vi "get-stage-positions.vi"(8 "error in (no error)":errorcluster, 11 "Cluster":T2) -> (0 "error out":errorcluster, 3 "stage positions":T1)   [LabVIEW 2024]
uses:
  C:/Users/hpDIRC/Desktop/eic_dirc_daq-LabVIEW_new/Thorlabs/Thorlabs.MotionControl.IntegratedStepperMotorsCLI.dll
  Thorlabs/Thorlabs.MotionControl.IntegratedStepperMotorsCLI.dll
  C:/Users/hpDIRC/Desktop/eic_dirc_daq-LabVIEW_new/Thorlabs/Thorlabs.MotionControl.Benchtop.StepperMotorCLI.dll
  Thorlabs/Thorlabs.MotionControl.Benchtop.StepperMotorCLI.dll
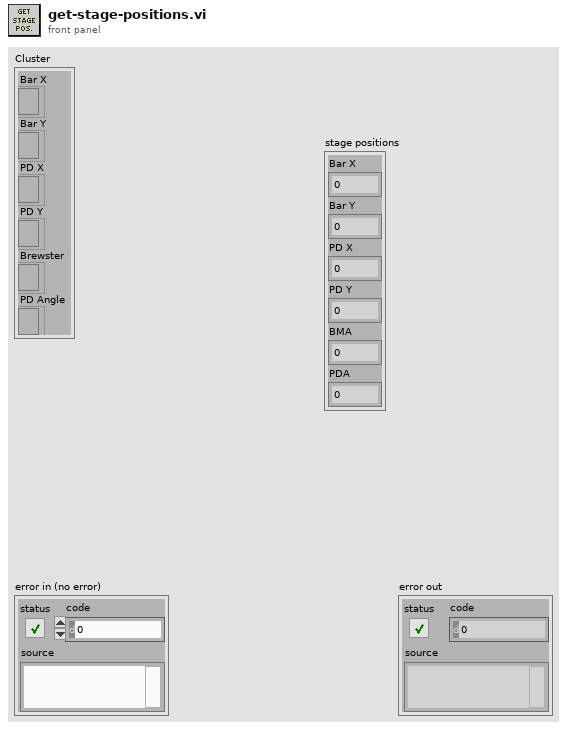
[diagram p1: front panel]
types:
  T1 = cluster{"Bar X":dbl, "Bar Y":dbl, "PD X":dbl, "PD Y":dbl, "BMA":dbl, "PDA":dbl}
  T2 = cluster{"Bar X":refnum<k24>, "Bar Y":refnum<k24>, "PD X":refnum<k24>, "PD Y":refnum<k24>, "Brewster":refnum<k24>, "PD Angle":refnum<k24>}
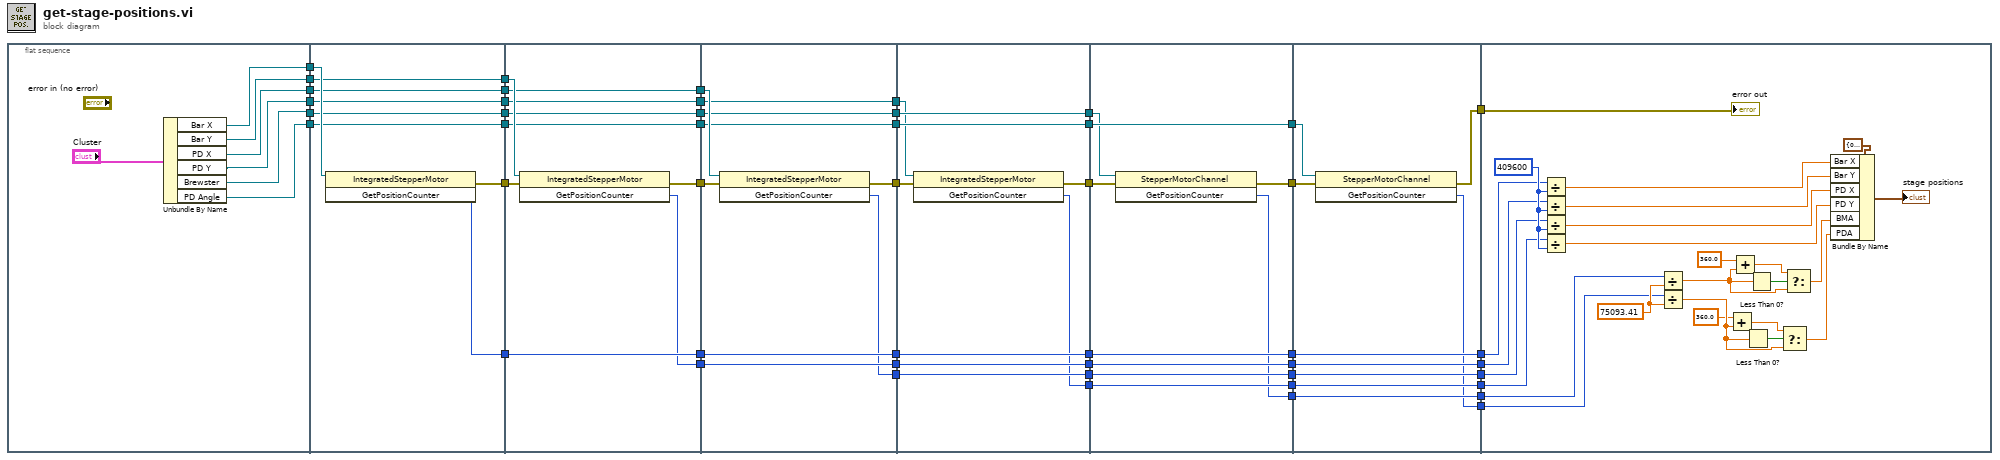
[diagram p0: block diagram]
diagram:
  n1 = flat-sequence {
    tunnel: [w54] -> w48
    tunnel: [w53] -> w45
    tunnel: [w52] -> w40
    tunnel: [w51] -> w39
    tunnel: [w50] -> w38
    tunnel: [w49] -> w37
    tunnel: [w62] -> w47
    tunnel: w48 -> [w63]
    tunnel: [w61] -> w46
    tunnel: w45 -> [w61]
    tunnel: [w60] -> w41
    tunnel: w40 -> [w60]
    tunnel: w39 -> [w59]
    tunnel: w38 -> [w58]
    tunnel: w37 -> [w57]
    tunnel: [w59] -> w36
    tunnel: [w58] -> w35
    tunnel: [w57] -> w34
    tunnel: [w56] -> w6
    tunnel: [w70] -> w44
    tunnel: w47 -> [w72]
    tunnel: [w72] -> w43
    tunnel: w46 -> [w71]
    tunnel: [w69] -> w42
    tunnel: w41 -> [w69]
    tunnel: w36 -> [w68]
    tunnel: w35 -> [w67]
    tunnel: w34 -> [w66]
    tunnel: [w68] -> w33
    tunnel: [w67] -> w32
    tunnel: [w66] -> w31
    tunnel: w6 -> [w65]
    tunnel: [w64] -> w5
    tunnel: [w78] -> w30
    tunnel: w44 -> [w81]
    tunnel: [w81] -> w29
    tunnel: w43 -> [w80]
    tunnel: [w80] -> w28
    tunnel: w42 -> [w79]
    tunnel: w33 -> [w75]
    tunnel: [w77] -> w27
    tunnel: w32 -> [w77]
    tunnel: [w76] -> w26
    tunnel: w31 -> [w76]
    tunnel: [w75] -> w25
    tunnel: w5 -> [w74]
    tunnel: [w73] -> w4
    tunnel: [w84] -> w24
    tunnel: w30 -> [w90]
    tunnel: [w90] -> w23
    tunnel: w29 -> [w89]
    tunnel: [w89] -> w22
    tunnel: w28 -> [w88]
    tunnel: [w88] -> w21
    tunnel: w27 -> [w87]
    tunnel: [w87] -> w20
    tunnel: w26 -> [w86]
    tunnel: [w86] -> w19
    tunnel: w25 -> [w85]
    tunnel: w4 -> [w83]
    tunnel: [w82] -> w3
    tunnel: [w93] -> w17
    tunnel: w24 -> [w99]
    tunnel: [w99] -> w15
    tunnel: w23 -> [w98]
    tunnel: [w98] -> w13
    tunnel: w22 -> [w97]
    tunnel: [w97] -> w11
    tunnel: w21 -> [w96]
    tunnel: [w96] -> w9
    tunnel: w20 -> [w94]
    tunnel: w19 -> [w95]
    tunnel: [w95] -> w7
    tunnel: w3 -> [w92]
    tunnel: [w91] -> w2
    tunnel: [w102] -> w18
    tunnel: w17 -> [w108]
    tunnel: [w108] -> w16
    tunnel: w15 -> [w107]
    tunnel: [w107] -> w14
    tunnel: w13 -> [w106]
    tunnel: [w106] -> w12
    tunnel: w11 -> [w105]
    tunnel: [w105] -> w10
    tunnel: w9 -> [w104]
    tunnel: [w104] -> w8
    tunnel: w7 -> [w103]
    tunnel: w2 -> [w101]
    tunnel: [w100] -> w1
    tunnel: w18 -> [w120]
    tunnel: w16 -> [w119]
    tunnel: w14 -> [w110]
    tunnel: w12 -> [w117]
    tunnel: w10 -> [w116]
    tunnel: w8 -> [w115]
    tunnel: w1 -> [w109]
    frame #0 {
      n2 = Unbundle By Name("Cluster") -> ("Bar X"=w54:refnum<k24>, "Bar Y"=w53:refnum<k24>, "PD X"=w52:refnum<k24>, "PD Y"=w51:refnum<k24>, "Brewster"=w50:refnum<k24>, "PD Angle"=w49:refnum<k24>)
    }
    frame #1 {
      n3 = invoke class="IntegratedStepperMotor" method="GetPositionCounter"(reference=w63) -> (error out=w56:errorcluster, "GetPositionCounter"=w62:i32)  [unwired: 2 in, 1 out]
    }
    frame #2 {
      n4 = invoke class="IntegratedStepperMotor" method="GetPositionCounter"(reference=w71, error in=w65) -> (error out=w64:errorcluster, "GetPositionCounter"=w70:i32)  [unwired: 1 in, 1 out]
    }
    frame #3 {
      n5 = invoke class="IntegratedStepperMotor" method="GetPositionCounter"(reference=w79, error in=w74) -> (error out=w73:errorcluster, "GetPositionCounter"=w78:i32)  [unwired: 1 in, 1 out]
    }
    frame #4 {
      n6 = invoke class="IntegratedStepperMotor" method="GetPositionCounter"(reference=w85, error in=w83) -> (error out=w82:errorcluster, "GetPositionCounter"=w84:i32)  [unwired: 1 in, 1 out]
    }
    frame #5 {
      n7 = invoke class="StepperMotorChannel" method="GetPositionCounter"(reference=w94, error in=w92) -> (error out=w91:errorcluster, "GetPositionCounter"=w93:i32)  [unwired: 1 in, 1 out]
    }
    frame #6 {
      n8 = invoke class="StepperMotorChannel" method="GetPositionCounter"(reference=w103, error in=w101) -> (error out=w100:errorcluster, "GetPositionCounter"=w102:i32)  [unwired: 1 in, 1 out]
    }
    frame #7 {
      w118 = 409600 ("y")
      w121 = 75093.41 ("GetPositionCounter")
      n9 = Divide(x=w115, y=w118) -> (x/y=w111:dbl)
      n10 = Divide(x=w116, y=w118) -> (x/y=w112:dbl)
      n11 = Divide(x=w117, y=w118) -> (x/y=w113:dbl)
      n12 = Divide(x=w110, y=w118) -> (x/y=w114:dbl)
      n13 = Divide(x=w119, y=w121) -> (x/y=w130:dbl)
      n14 = Divide(x=w120, y=w121) -> (x/y=w126:dbl)
      n15 = Add(x=360.0, y=w126) -> (x+y=w128:dbl)
      n16 = Add(x=360.0, y=w130) -> (x+y=w129:dbl)
      n17 = Less Than 0?(x=w126) -> (x < 0?=w127:bool)
      n18 = Less Than 0?(x=w130) -> (x < 0?=w131:bool)
      n19 = Select(t=w128, s=w127, f=w126) -> (s? t:f=w133:dbl)
      n20 = Select(t=w129, s=w131, f=w130) -> (s? t:f=w132:dbl)
      n21 = Bundle By Name(cluster=T1 {"Bar X"=0.0, "Bar Y"=0.0, "PD X"=0.0, "PD Y"=0.0, "BMA"=0.0, "PDA"=0.0} ("stage positions 2"), "Bar X"=w111, "Bar Y"=w112, "PD X"=w113, "PD Y"=w114, "BMA"=w132, "PDA"=w133) -> (→"stage positions":T1)
      "error out" <- w109
    }
  }
